vi "Send TCP Request and Wait on Response.vi"(6 "Timeout (ms)":u32, 8 "error in (no error)":errorcluster, 9 "Data":string, 10 "Name":string, 11 "Connection Info":T1) -> (0 "error out":errorcluster, 1 "Data":string, 2 "Timed Out?":bool, 3 "Connection Info Out":T1)   [LabVIEW 2013, in "PID Control Host API.lvlib"]
uses:
  <userlib>/STM/TCP/stm_TCP Connection Info.ctl
  <userlib>/STM/_SubVIs/stm_MetaDataElement.ctl
  <userlib>/STM/TCP/stm_TCP Read Options.ctl
  <userlib>/STM/TCP/STM Write Message (TCP).vi
  <userlib>/STM/TCP/STM Read Message (TCP).vi
  PID Control Host API.lvlib
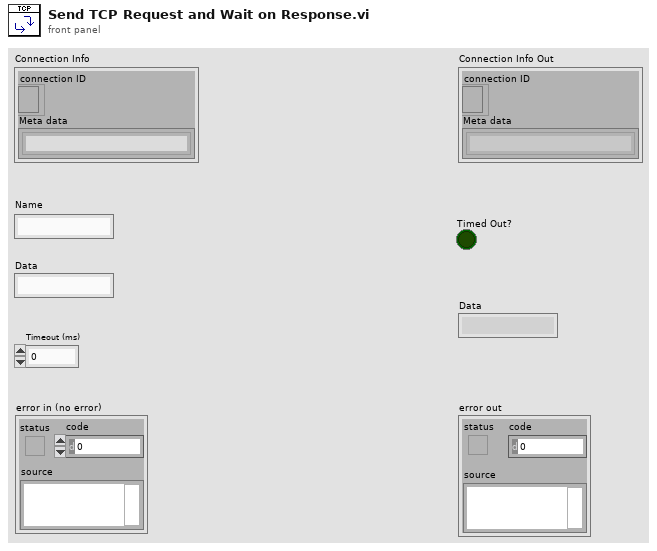
[diagram p1: front panel]
types:
  T1 = typedef "stm_TCP Connection Info.ctl" = cluster{"connection ID":refnum<k5>, "Meta data":T2[]}
  T2 = typedef "stm_MetaDataElement.ctl" = string
  T3 = typedef "stm_TCP Read Options.ctl" = cluster{"Ignore Timeout Error":bool, "timeout ms (1000)":i32}
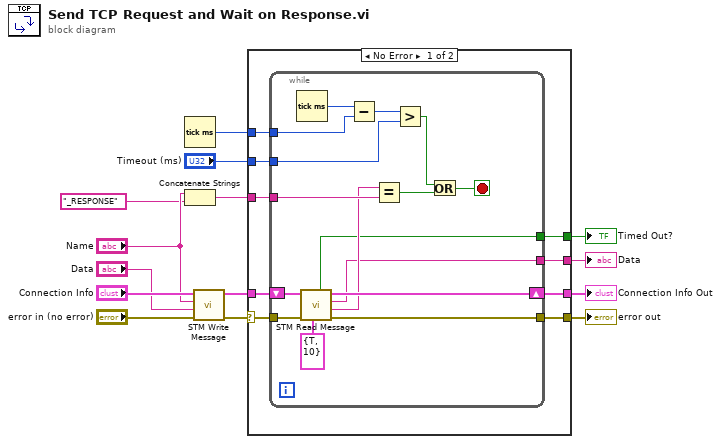
[diagram p0: block diagram]
diagram:
  n1 = Tick Count (ms)() -> (millisecond timer value=w6:u32)
  n2 = Concatenate Strings("Name", "_RESPONSE" ("string")) -> (w7:string)
  n3 = call-poly <userlib>:"STM Write Message.vi"("error in (no error)"="error in (no error)", "Data"="Data", "Name"="Name", "Connection Info"="Connection Info") -> ("error out"=w1:errorcluster, "Connection Info Out"=w14:T1)  [unwired: 6 in]
  n4 = case shown="No Error" w1 {
    selector: w1 -> [w15 w41]
    tunnel: w14 -> [w23 w40]
    tunnel: [w22 w41] -> w10
    tunnel: w7 -> [w21 _]
    tunnel: w6 -> [w20 _]
    tunnel: "Timeout (ms)" -> [w19 _]
    tunnel: [w18 w40] -> w4
    tunnel: [w17 _] -> w3
    tunnel: [w16 _] -> w2
    frame No Error {
      n5 = while {
        tunnel: w15 -> [w38]
        tunnel: [w37] -> w22
        tunnel: w21 -> [w36]
        tunnel: w20 -> [w34]
        tunnel: w19 -> [w32]
        shift-right: [w28] -> w18
        shift-left: w23 -> [w39]
        tunnel: [w26] -> w17
        tunnel: [w25] -> w16
        stop <- w29 stop-if-true
        n6 = Tick Count (ms)() -> (millisecond timer value=w35:u32)
        n7 = call-poly <userlib>:"STM Read Message.vi"("Options"=T3 {"Ignore Timeout Error"=TRUE, "timeout ms (1000)"=10}, "error in"=w38, "Connection Info"=w39) -> ("error out"=w37:errorcluster, "Name"=w27:T2, "data string"=w26:string, "Connection Info Out"=w28:T1, "Timed Out?"=w25:bool)  [unwired: 3 in, 1 out]
        n8 = Subtract(x=w35, y=w34) -> (x-y=w33:u32)
        n9 = Equal?(x=w27, y=w36) -> (x = y?=w30:bool)
        n10 = Greater?(x=w33, y=w32) -> (0:w31:bool)
        n11 = Or(x=w31, y=w30) -> (x .or. y?=w29:bool)
      }
    }
    frame Error {
    }
  }
  "error out" <- w10
  "Connection Info Out" <- w4
  "Data" <- w3
  "Timed Out?" <- w2
